vi "Write DisabledTime.vi"(8 "error in (no error)":errorcluster, 10 "DisabledTime":dbl, 11 "SnakeSwitch in":refnum<class "SnakeSwitch.lvclass">) -> (0 "error out":errorcluster, 3 "SnakeSwitch out":refnum<class "SnakeSwitch.lvclass">)   [LabVIEW 2019, in "RT_Game.lvlib" / "SnakeSwitch.lvclass"]
uses:
  SnakeSwitch.lvclass
  SnakeSwitch.lvclass/SnakeSwitch.ctl
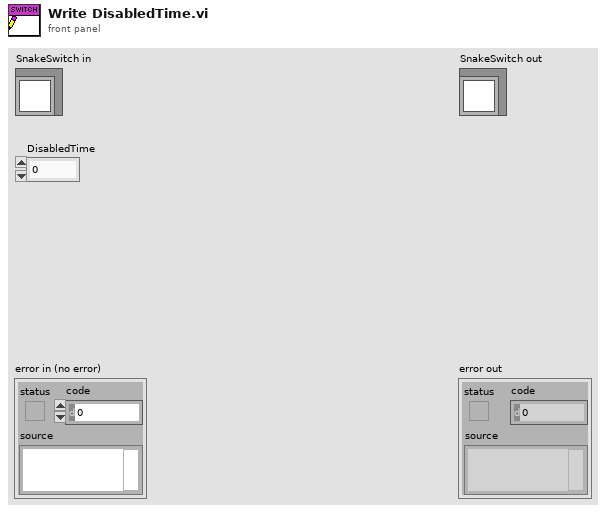
[diagram p1: front panel]
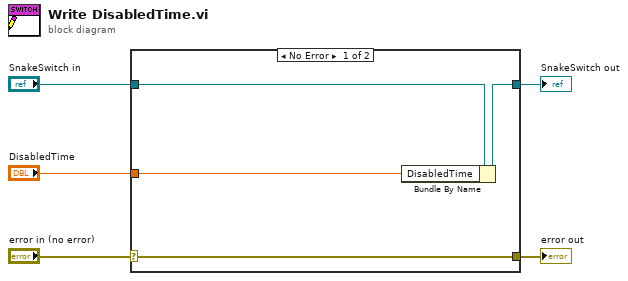
[diagram p0: block diagram]
diagram:
  n1 = case shown="No Error" "error in (no error)" {
    selector: "error in (no error)" -> [w9 w10]
    tunnel: [w9 w10] -> w4
    tunnel: [w7 w11] -> w2
    tunnel: "SnakeSwitch in" -> [w8 w11]
    tunnel: "DisabledTime" -> [w6 _]
    frame No Error {
      n2 = Bundle By Name(cluster=w8, "DisabledTime"=w6) -> (w7:refnum<class "SnakeSwitch.lvclass">)
    }
    frame Error {
    }
  }
  "error out" <- w4
  "SnakeSwitch out" <- w2
